vi "Destroy User Events.vi"(11 "UI Template in":refnum<class "Laser Oxxius Controller.lvclass">) -> (3 "UI Template out":refnum<class "Laser Oxxius Controller.lvclass">)   [LabVIEW 2020, in "Laser_Oxxius.lvlib" / "Laser Oxxius Controller.lvlib" / "Laser Oxxius Controller.lvclass"]
uses:
  Laser Oxxius Controller.lvclass
  Laser Oxxius Controller.lvclass/Laser Oxxius Controller.ctl
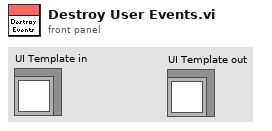
[diagram p1: front panel]
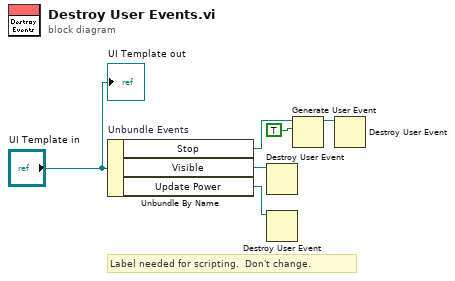
[diagram p0: block diagram]
diagram:
  # "Label needed for scripting.  Don't change."
  n1 = Unbundle By Name "Unbundle Events"("UI Template in") -> ("Stop"=w4:refnum<user-event>, "Visible"=w2:refnum<user-event>, "Update Power"=w1:refnum<user-event>)
  n2 = Destroy User Event(user event=w2) -> ()  [unwired: 1 in, 1 out]
  n3 = Destroy User Event(user event=w1) -> ()  [unwired: 1 in, 1 out]
  n4 = Generate User Event(user event=w4, event data cluster=TRUE ("event data")) -> (user event out=w5:refnum<user-event>)  [unwired: 2 in, 1 out]
  n5 = Destroy User Event(user event=w5) -> ()  [unwired: 1 in, 1 out]
  "UI Template out" <- "UI Template in"
